vi "RT_Control_Adrian_Microphones+Angles+Force_NoPower.vi"(10 "rt fifo":refnum<k33>, 11 "Parameters":T1={"N_chan"=0, "Input Rate (Hz)"=0.0, "Acq Time (s)"=0.0, "NumOfWarmupIters"=0, "Size fifo"=0, "Period NCL (ms)"=0, "Timeout fifo Read"=0, "Size Sent Array"=0, "Output offsets"=[], "Input offsets"=[0.0, 0.0, 0.0, 0.0, 0.0, 0.0, 0.0, 0.0]}) -> (0 "error out":errorcluster, 1 "Total Iterations":i64, 2 "Delayed Cycles":dbl)   [LabVIEW 2021]
uses:
  parametersRT.ctl
  <vilib>/DAQmx/write.llb/DAQmx Write (Analog 1D DBL NChan 1Samp).vi
  <vilib>/DAQmx/read.llb/DAQmx Read (Analog 1D DBL NChan 1Samp).vi
  <vilib>/Analysis/baseanly.llb/A x Vector.vi
  <vilib>/DAQmx/read.llb/DAQmx Read (Digital 2D U32 NChan NSamp).vi
  <vilib>/Analysis/baseanly.llb/Mean (DBL).vi
  <vilib>/DAQmx/configure/timing.llb/DAQmx Timing (Sample Clock).vi
  <vilib>/DAQmx/miscellaneous.llb/DAQmx Fill In Error Info.vi
  <resource>/objmgr/daqmx.rc
  <vilib>/Analysis/NI_AALBase.lvlib
panel:
  out "output array":dbl[](array[numeric])
  out "data 2":u32[][](array[numeric])
  out "Encoder Raw Outputs":dbl[][](array[numeric])
  out "Encoder Mean Outputs":dbl[](array[numeric])
  in  "Zero Angle":dbl[](array[numeric])=[-16.79, 2.64, -15.0, 3.7]
  in  "source 2":tag
  in  "source":tag
  out "A x Vector":dbl[](array[numeric]) format="%.2f"
  in  "Unbias":bool
  out "Bias Voltages":dbl[][](array[numeric])=[[-0.0710179470114859, -0.17463349299050945, -0.11016159714741332, 0.026018829634351103, 0.12897648926553976, 0.08259620236774425]]
  out "Bias Vector":dbl[](array[numeric])=[-0.0710179470114859, -0.17463349299050945, -0.11016159714741332, 0.026018829634351103, 0.12897648926553976, 0.08259620236774425]
  in  "Bias":bool
  out "Voltages":dbl[][](array[numeric])=[[-0.07200476171213811, -0.17430455474177844, -0.11114841186574954, 0.027005644288728526, 0.12535816905124034, 0.08062257311350753], [-0.07233369994578917, -0.17397561649309423, -0.11147735010529275, 0.027334582506747616, 0.1263449836558195, 0.08160938774087402], [-0.0716758234785372, -0.17463349299050945, -0.11147735010529275, 0.026676706070656076, 0.1260160454543497, 0.08062257311350753], [-0.07200476171213811, -0.1749624312392873, -0.1118062883448848, 0.026676706070656076, 0.1256871072528233, 0.08029363490427514], [-0.07200476171213811, -0.17430455474177844, -0.11213522658452575, 0.026676706070656076, 0.12535816905124034, 0.08029363490427514], [-0.07233369994578917, -0.1749624312392873, -0.11147735010529275, 0.027334582506747616, 0.1260160454543497, 0.08062257311350753], [-0.07200476171213811, -0.17397561649309423, -0.11147735010529275, 0.027005644288728526, 0.1260160454543497, 0.08029363490427514], [-0.07200476171213811, -0.17463349299050945, -0.1118062883448848, 0.027005644288728526, 0.1260160454543497, 0.08062257311350753], [-0.07233369994578917, -0.17397561649309423, -0.11114841186574954, 0.027334582506747616, 0.1263449836558195, 0.08062257311350753], [-0.07233369994578917, -0.17463349299050945, -0.1118062883448848, 0.026676706070656076, 0.1256871072528233, 0.08029363490427514], [-0.07200476171213811, -0.17463349299050945, -0.11213522658452575, 0.027334582506747616, 0.1256871072528233, 0.08062257311350753], [-0.07233369994578917, -0.17463349299050945, -0.1118062883448848, 0.027005644288728526, 0.1256871072528233, 0.08029363490427514], [-0.07200476171213811, -0.17463349299050945, -0.1118062883448848, 0.027334582506747616, 0.1260160454543497, 0.08029363490427514], [-0.0716758234785372, -0.17430455474177844, -0.11147735010529275, 0.027334582506747616, 0.1263449836558195, 0.08128044953180698], [-0.07200476171213811, -0.17463349299050945, -0.11114841186574954, 0.027005644288728526, 0.1263449836558195, 0.08029363490427514], [-0.07266263817949037, -0.17430455474177844, -0.11213522658452575, 0.027005644288728526, 0.1256871072528233, 0.08029363490427514], [-0.07233369994578917, -0.17463349299050945, -0.1118062883448848, 0.027334582506747616, 0.1263449836558195, 0.08128044953180698], [-0.07200476171213811, -0.17397561649309423, -0.1118062883448848, 0.026676706070656076, 0.1260160454543497, 0.08029363490427514], [-0.07233369994578917, -0.17397561649309423, -0.11147735010529275, 0.027334582506747616, 0.1263449836558195, 0.08128044953180698], [-0.0716758234785372, -0.17397561649309423, -0.11147735010529275, 0.027334582506747616, 0.1256871072528233, 0.08029363490427514], [-0.07200476171213811, -0.17430455474177844, -0.1118062883448848, 0.027334582506747616, 0.1263449836558195, 0.08095151132268481], [-0.07266263817949037, -0.17463349299050945, -0.1118062883448848, 0.026676706070656076, 0.1260160454543497, 0.08029363490427514], [-0.07200476171213811, -0.1736466782444569, -0.1118062883448848, 0.027005644288728526, 0.12535816905124034, 0.08095151132268481], [-0.07233369994578917, -0.1749624312392873, -0.11147735010529275, 0.027005644288728526, 0.1263449836558195, 0.08062257311350753], [-0.07200476171213811, -0.1736466782444569, -0.11114841186574954, 0.02766352072471333, 0.1263449836558195, 0.08062257311350753], [-0.07200476171213811, -0.17463349299050945, -0.1118062883448848, 0.027005644288728526, 0.1256871072528233, 0.08029363490427514], [-0.07266263817949037, -0.17430455474177844, -0.11213522658452575, 0.027334582506747616, 0.1260160454543497, 0.08062257311350753], [-0.07200476171213811, -0.17430455474177844, -0.11147735010529275, 0.02766352072471333, 0.1263449836558195, 0.08062257311350753], [-0.07200476171213811, -0.1749624312392873, -0.11213522658452575, 0.027334582506747616, 0.1260160454543497, 0.08062257311350753], [-0.07233369994578917, -0.17430455474177844, -0.11147735010529275, 0.027334582506747616, 0.1260160454543497, 0.08029363490427514], [-0.07233369994578917, -0.17397561649309423, -0.1118062883448848, 0.027334582506747616, 0.1263449836558195, 0.08062257311350753], [-0.0716758234785372, -0.17397561649309423, -0.11213522658452575, 0.027334582506747616, 0.1260160454543497, 0.07996469669498764], [-0.07266263817949037, -0.17430455474177844, -0.1118062883448848, 0.02766352072471333, 0.1263449836558195, 0.08062257311350753], [-0.07266263817949037, -0.17430455474177844, -0.1118062883448848, 0.027334582506747616, 0.1256871072528233, 0.08029363490427514], [-0.07200476171213811, -0.17463349299050945, -0.1118062883448848, 0.026676706070656076, 0.12535816905124034, 0.07963575848564507], [-0.07233369994578917, -0.17397561649309423, -0.11114841186574954, 0.02766352072471333, 0.1263449836558195, 0.08062257311350753], [-0.07266263817949037, -0.1749624312392873, -0.11213522658452575, 0.026676706070656076, 0.12535816905124034, 0.07963575848564507], [-0.07233369994578917, -0.17463349299050945, -0.1118062883448848, 0.027005644288728526, 0.1256871072528233, 0.07996469669498764], [-0.07299157641324171, -0.17463349299050945, -0.11213522658452575, 0.026676706070656076, 0.1260160454543497, 0.08029363490427514], [-0.07233369994578917, -0.17430455474177844, -0.11147735010529275, 0.027334582506747616, 0.12667392185723272, 0.08095151132268481], [-0.07200476171213811, -0.1736466782444569, -0.11147735010529275, 0.02766352072471333, 0.1263449836558195, 0.08062257311350753], [-0.07233369994578917, -0.17397561649309423, -0.1118062883448848, 0.026676706070656076, 0.1260160454543497, 0.07996469669498764], [-0.07233369994578917, -0.17463349299050945, -0.11213522658452575, 0.027005644288728526, 0.1260160454543497, 0.08029363490427514], [-0.07200476171213811, -0.17331773999586642, -0.11081947362625524, 0.02766352072471333, 0.12667392185723272, 0.08095151132268481], [-0.07233369994578917, -0.17397561649309423, -0.1118062883448848, 0.02766352072471333, 0.1260160454543497, 0.08029363490427514], [-0.07266263817949037, -0.17463349299050945, -0.11213522658452575, 0.02766352072471333, 0.1260160454543497, 0.08128044953180698], [-0.07200476171213811, -0.17397561649309423, -0.11147735010529275, 0.02766352072471333, 0.1263449836558195, 0.08095151132268481], [-0.07200476171213811, -0.17430455474177844, -0.1118062883448848, 0.027334582506747616, 0.1263449836558195, 0.08095151132268481], [-0.0716758234785372, -0.17463349299050945, -0.1118062883448848, 0.027005644288728526, 0.1263449836558195, 0.08095151132268481], [-0.07200476171213811, -0.17397561649309423, -0.1118062883448848, 0.027005644288728526, 0.1256871072528233, 0.08029363490427514], [-0.07233369994578917, -0.17430455474177844, -0.11147735010529275, 0.027334582506747616, 0.1263449836558195, 0.08095151132268481], [-0.0716758234785372, -0.1736466782444569, -0.11114841186574954, 0.027992458942625646, 0.12667392185723272, 0.08095151132268481], [-0.07200476171213811, -0.17397561649309423, -0.1118062883448848, 0.027334582506747616, 0.1263449836558195, 0.08029363490427514], [-0.07200476171213811, -0.17397561649309423, -0.11114841186574954, 0.027334582506747616, 0.1263449836558195, 0.08029363490427514], [-0.07233369994578917, -0.17397561649309423, -0.1118062883448848, 0.027334582506747616, 0.1260160454543497, 0.08029363490427514], [-0.07266263817949037, -0.17430455474177844, -0.11213522658452575, 0.026676706070656076, 0.1260160454543497, 0.08029363490427514], [-0.07233369994578917, -0.17397561649309423, -0.11213522658452575, 0.027334582506747616, 0.1263449836558195, 0.08062257311350753], [-0.07233369994578917, -0.17463349299050945, -0.11213522658452575, 0.027334582506747616, 0.1260160454543497, 0.08029363490427514], [-0.07200476171213811, -0.17331773999586642, -0.11147735010529275, 0.027334582506747616, 0.1263449836558195, 0.08029363490427514], [-0.07233369994578917, -0.1749624312392873, -0.11213522658452575, 0.026676706070656076, 0.1260160454543497, 0.08029363490427514], [-0.07233369994578917, -0.17463349299050945, -0.1118062883448848, 0.027005644288728526, 0.1260160454543497, 0.08029363490427514], [-0.07233369994578917, -0.17397561649309423, -0.1118062883448848, 0.027334582506747616, 0.12667392185723272, 0.08062257311350753], [-0.07200476171213811, -0.17430455474177844, -0.11147735010529275, 0.027334582506747616, 0.1260160454543497, 0.07996469669498764], [-0.07233369994578917, -0.17430455474177844, -0.1118062883448848, 0.027334582506747616, 0.12667392185723272, 0.08095151132268481], [-0.0716758234785372, -0.17430455474177844, -0.11147735010529275, 0.026676706070656076, 0.1263449836558195, 0.08029363490427514], [-0.07266263817949037, -0.17430455474177844, -0.11147735010529275, 0.027005644288728526, 0.1263449836558195, 0.07996469669498764], [-0.07266263817949037, -0.1749624312392873, -0.11246416482421552, 0.026676706070656076, 0.1263449836558195, 0.08029363490427514], [-0.07266263817949037, -0.17397561649309423, -0.1118062883448848, 0.027334582506747616, 0.1263449836558195, 0.08029363490427514], [-0.0716758234785372, -0.1736466782444569, -0.11147735010529275, 0.02766352072471333, 0.1263449836558195, 0.08062257311350753], [-0.07233369994578917, -0.17397561649309423, -0.1118062883448848, 0.027334582506747616, 0.1263449836558195, 0.08095151132268481], [-0.07233369994578917, -0.17430455474177844, -0.1118062883448848, 0.027334582506747616, 0.1260160454543497, 0.08062257311350753], [-0.0716758234785372, -0.17331773999586642, -0.11081947362625524, 0.027992458942625646, 0.12700286005858935, 0.08062257311350753], [-0.07233369994578917, -0.17397561649309423, -0.11213522658452575, 0.027005644288728526, 0.1263449836558195, 0.08029363490427514], [-0.07233369994578917, -0.17463349299050945, -0.11147735010529275, 0.027005644288728526, 0.1260160454543497, 0.08029363490427514], [-0.07266263817949037, -0.1736466782444569, -0.11147735010529275, 0.02766352072471333, 0.12667392185723272, 0.08029363490427514], [-0.07200476171213811, -0.17463349299050945, -0.11213522658452575, 0.026676706070656076, 0.1260160454543497, 0.07996469669498764], [-0.07266263817949037, -0.17430455474177844, -0.11213522658452575, 0.027005644288728526, 0.1263449836558195, 0.08062257311350753], [-0.07200476171213811, -0.17397561649309423, -0.11147735010529275, 0.02766352072471333, 0.1263449836558195, 0.08062257311350753], [-0.07200476171213811, -0.17397561649309423, -0.1118062883448848, 0.027005644288728526, 0.1263449836558195, 0.08029363490427514], [-0.07233369994578917, -0.17430455474177844, -0.11213522658452575, 0.027005644288728526, 0.1263449836558195, 0.08062257311350753], [-0.07233369994578917, -0.1736466782444569, -0.11114841186574954, 0.027334582506747616, 0.12667392185723272, 0.08062257311350753], [-0.07233369994578917, -0.17430455474177844, -0.1118062883448848, 0.027334582506747616, 0.1260160454543497, 0.08029363490427514], [-0.07266263817949037, -0.17529136948811197, -0.11279310306395414, 0.026676706070656076, 0.1263449836558195, 0.08029363490427514], [-0.07233369994578917, -0.17397561649309423, -0.11147735010529275, 0.027005644288728526, 0.12667392185723272, 0.08062257311350753], [-0.07200476171213811, -0.17430455474177844, -0.1118062883448848, 0.027334582506747616, 0.1263449836558195, 0.07996469669498764], [-0.07233369994578917, -0.17463349299050945, -0.11246416482421552, 0.027005644288728526, 0.1256871072528233, 0.07996469669498764], [-0.07266263817949037, -0.17430455474177844, -0.1118062883448848, 0.026676706070656076, 0.1260160454543497, 0.07996469669498764], [-0.07266263817949037, -0.17463349299050945, -0.1118062883448848, 0.027005644288728526, 0.1260160454543497, 0.08062257311350753], [-0.07266263817949037, -0.17397561649309423, -0.1118062883448848, 0.02766352072471333, 0.1263449836558195, 0.07996469669498764], [-0.07233369994578917, -0.17463349299050945, -0.1118062883448848, 0.027005644288728526, 0.1260160454543497, 0.08062257311350753], [-0.0716758234785372, -0.17397561649309423, -0.11114841186574954, 0.02766352072471333, 0.12667392185723272, 0.08095151132268481], [-0.07200476171213811, -0.17430455474177844, -0.11147735010529275, 0.027005644288728526, 0.1260160454543497, 0.08029363490427514], [-0.07200476171213811, -0.17397561649309423, -0.11114841186574954, 0.027992458942625646, 0.12700286005858935, 0.08128044953180698], [-0.07134688524498646, -0.17397561649309423, -0.1118062883448848, 0.027005644288728526, 0.1263449836558195, 0.07996469669498764], [-0.07266263817949037, -0.17463349299050945, -0.11213522658452575, 0.026676706070656076, 0.1256871072528233, 0.07996469669498764], [-0.07266263817949037, -0.17430455474177844, -0.11147735010529275, 0.027334582506747616, 0.12667392185723272, 0.08062257311350753], [-0.0716758234785372, -0.17463349299050945, -0.1118062883448848, 0.026676706070656076, 0.12667392185723272, 0.08029363490427514], [-0.07233369994578917, -0.17397561649309423, -0.1118062883448848, 0.027334582506747616, 0.1263449836558195, 0.08062257311350753], [-0.07233369994578917, -0.17463349299050945, -0.1118062883448848, 0.027005644288728526, 0.1260160454543497, 0.08029363490427514], [-0.07233369994578917, -0.17397561649309423, -0.11213522658452575, 0.027334582506747616, 0.1263449836558195, 0.08062257311350753]]
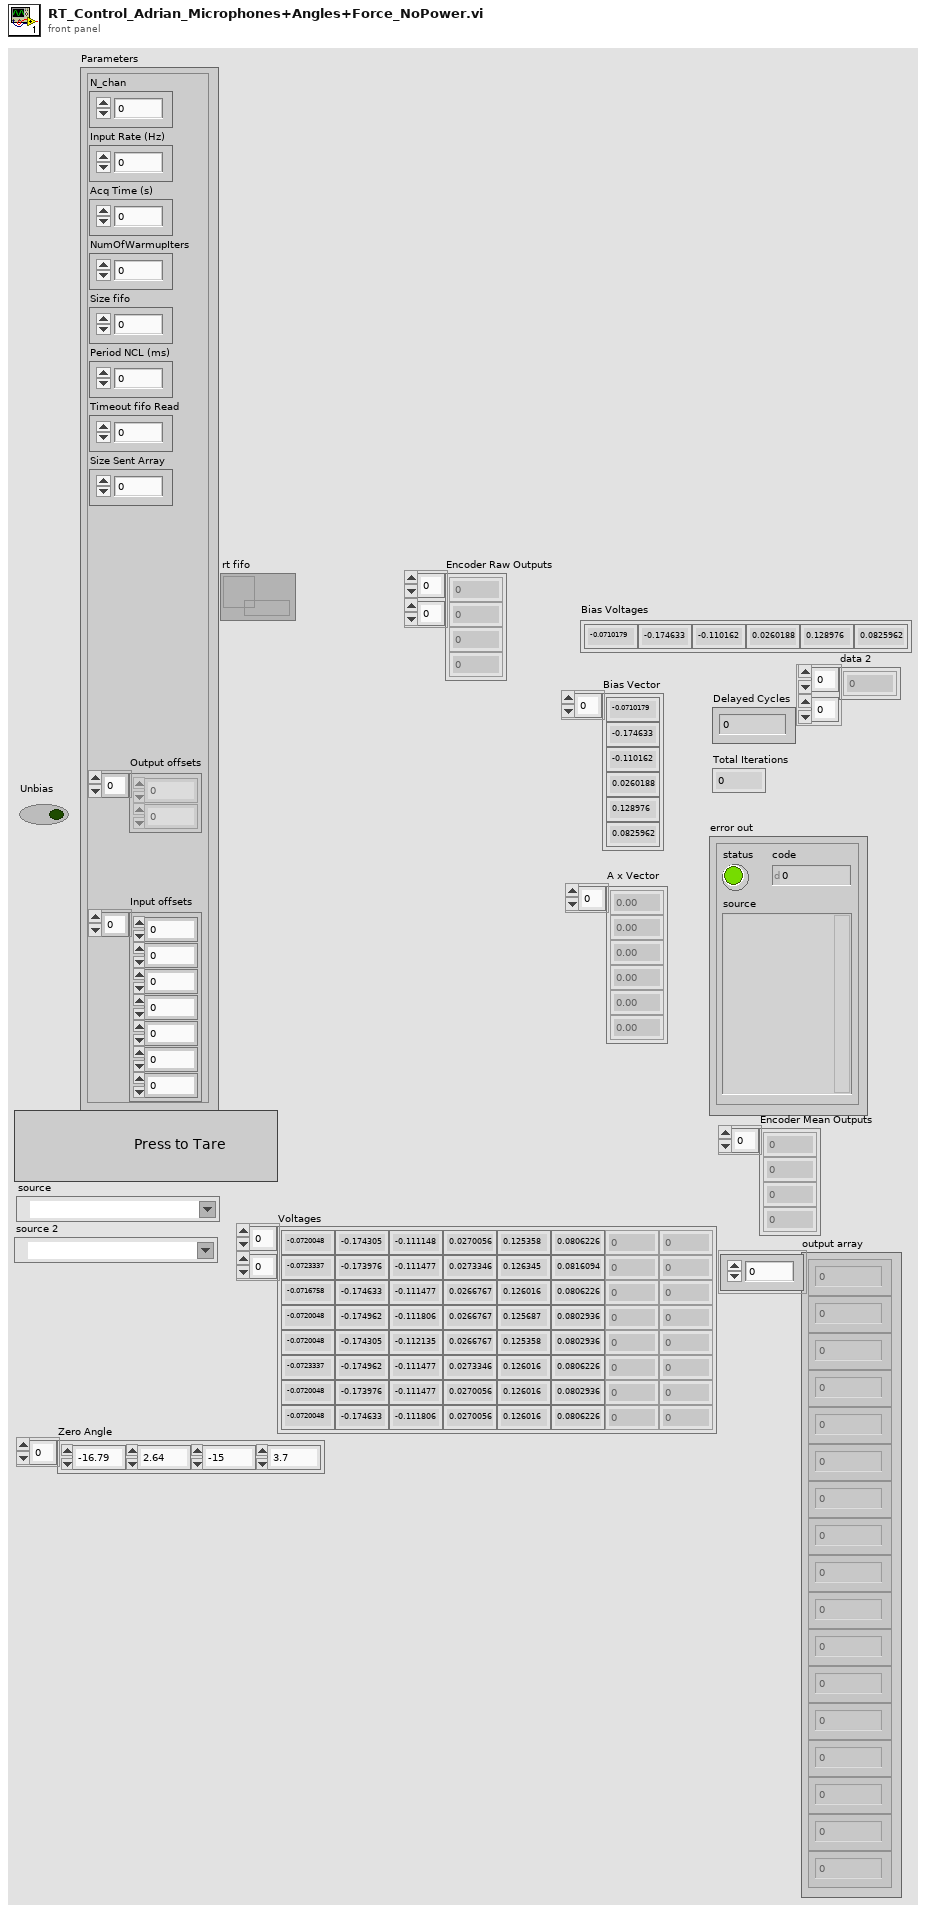
[diagram p1: front panel]
types:
  T1 = typedef "parametersRT.ctl" = cluster{"N_chan":u32, "Input Rate (Hz)":dbl, "Acq Time (s)":dbl, "NumOfWarmupIters":u32, "Size fifo":u32, "Period NCL (ms)":i64, "Timeout fifo Read":i32, "Size Sent Array":i32, "Output offsets":dbl[], "Input offsets":dbl[]}
  T2 = cluster{"Csn task out":refnum<k21>, "CLK task out":refnum<k21>, "D0 task out":refnum<k21>}
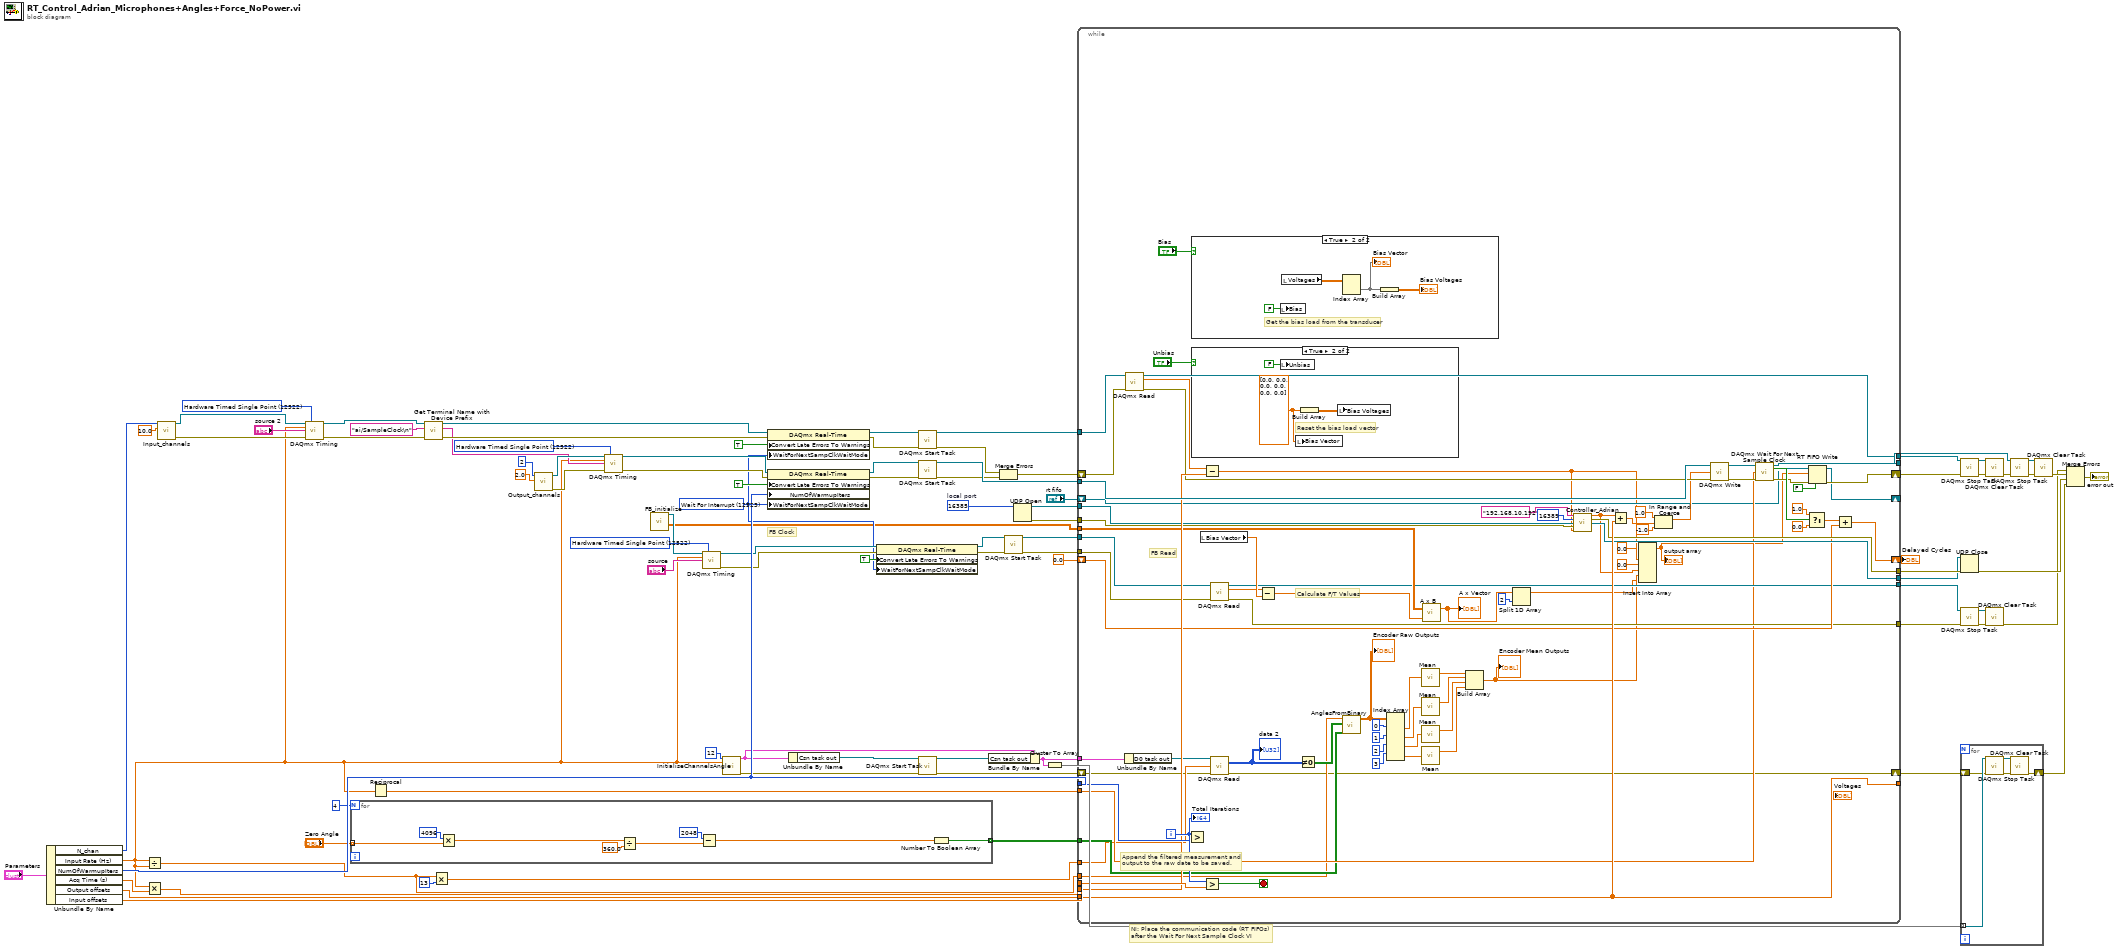
[diagram p0: block diagram]
diagram:
  w48 = 12522 items=["Finite Samples"=10178, "Continuous Samples"=10123, "Hardware Timed Single Point"=12522] ("sample mode")
  w59 = u16 16385  # local port
  w66 = 12522 items=["Finite Samples"=10178, "Continuous Samples"=10123, "Hardware Timed Single Point"=12522] ("sample mode")
  w43 = 12523 items=["Wait For Interrupt"=12523, "Poll"=12524, "Yield"=12525] ("WaitForNextSampClkWaitMode")
  w89 = 12522 items=["Finite Samples"=10178, "Continuous Samples"=10123, "Hardware Timed Single Point"=12522] ("sample mode")
  # "FB Clock"
  # "NI: Place the communication code (RT FIFOs) \nafter the Wait For Next Sample Clock VI"
  n1 = Unbundle By Name("Parameters") -> ("N_chan"=w75:u32, "Input Rate (Hz)"=w10:dbl, "NumOfWarmupIters"=w76:u32, "Acq Time (s)"=w83:dbl, "Output offsets"=w74:dbl[], "Input offsets"=w73:dbl[])
  n2 = Divide(x=w10, y=w10) -> (x/y=w8:dbl)
  n3 = Multiply(x=w10, y=w83) -> (x*y=w53:dbl)
  n4 = call "Input_channels.vi"("Range"=10.0, "nchan"=w75) -> ("error out"=w68:errorcluster, "Refnum out"=w67:refnum<k21>)  [unwired: 8 in]
  n5 = call-poly <vilib>:"DAQmx Timing.vi"("task/channels in"=w67, "sample mode"=w66, "rate"=w10, "source"="source 2", "error in"=w68) -> ("task out"=w36:refnum<k21>, "error out"=w34:errorcluster)  [unwired: 9 in]
  n6 = for {
    N: 4 -> [_]
    tunnel: [w94] -> w9 mode=indexing
    tunnel: "Zero Angle" -> [w97] mode=indexing
    n7 = Multiply(x=4096, y=w97) -> (x*y=w98:dbl)
    n8 = Divide(x=w98, y=360.0) -> (x/y=w92:dbl)
    n9 = Subtract(x=2048, y=w92) -> (x-y=w91:dbl)
    n10 = Number To Boolean Array(number=w91) -> (Boolean array=w94:bool[])
  }
  n11 = Reciprocal(x=w10) -> (1/x=w88:dbl)
  n12 = call "Get Terminal Name with Device Prefix.vi"("error in (no error)"=w34, "Local Terminal Name"="ai/SampleClock\n", "task/channels in"=w36) -> ("error out"=w33:errorcluster, "Terminal Name with Device Prefix"=w32:tag, "task out"=w35:refnum<k21>)  [unwired: 6 in]
  n13 = Multiply(x=w8, y=13) -> (x*y=w6:dbl)
  n14 = call "Output_channels.vi"("Range"=2.0 ("Maximum Value"), "nchan"=2) -> ("error out"=w80:errorcluster, "Refnum out"=w79:refnum<k21>)  [unwired: 8 in]
  n15 = call-poly <vilib>:"DAQmx Timing.vi"("task/channels in"=w79, "sample mode"=w89, "rate"=w10, "source"=w32, "error in"=w80) -> ("task out"=w87:refnum<k21>, "error out"=w86:errorcluster)  [unwired: 9 in]
  n16 = call "FB_initialize.vi"() -> ("Transformed Calibration Matrix"=w40:dbl[][], "FB out"=w44:refnum<k21>)  [unwired: 9 in, 1 out]
  n17 = call-poly <vilib>:"DAQmx Timing.vi"("task/channels in"=w44, "sample mode"=w48, "rate"=w10, "source"="source") -> ("task out"=w50:refnum<k21>, "error out"=w49:errorcluster)  [unwired: 10 in]
  n18 = call "InitialiseChannelsAngle.vi"("Number of data bits"=12, "Fs"=w10) -> ("output cluster"=w11:T2, "error out"=w12:errorcluster)  [unwired: 12 in]
  n19 = property class="DAQmx Real-Time"(reference=w35, error in=w33, "Convert Late Errors To Warnings"=TRUE, "WaitForNextSampClkWaitMode"=w43) -> (reference out=w63:refnum<k21>, error out=w62:errorcluster)
  n20 = property class="DAQmx Real-Time"(reference=w87, error in=w86, "Convert Late Errors To Warnings"=TRUE, "NumOfWarmupIters"=w76, "WaitForNextSampClkWaitMode"=w43) -> (reference out=w84:refnum<k21>, error out=w70:errorcluster)
  n21 = Unbundle By Name(w11) -> ("Csn task out"=w16:refnum<k21>)
  n22 = property class="DAQmx Real-Time"(reference=w50, error in=w49, "Convert Late Errors To Warnings"=TRUE ("ConvLateErrorsToWarnings"), "WaitForNextSampClkWaitMode"=w43) -> (reference out=w45:refnum<k21>, error out=w46:errorcluster)
  n23 = call <vilib>:"DAQmx Start Task.vi"("task/channels in"=w63, "error in"=w62) -> ("task out"=w82:refnum<k21>, "error out"=w61:errorcluster)  [unwired: 12 in]
  n24 = call <vilib>:"DAQmx Start Task.vi"("task/channels in"=w84, "error in"=w70) -> ("task out"=w81:refnum<k21>, "error out"=w69:errorcluster)  [unwired: 12 in]
  n25 = call <vilib>:"DAQmx Start Task.vi"("task/channels in"=w16, "error in"=w12) -> ("task out"=w15:refnum<k21>, "error out"=w3:errorcluster)  [unwired: 12 in]
  n26 = Bundle By Name(cluster=w11, "Csn task out"=w15) -> (w7:T2)
  n27 = Merge Errors(w61, w69) -> (w60:errorcluster)
  n28 = call <vilib>:"DAQmx Start Task.vi"("task/channels in"=w45, "error in"=w46) -> ("task out"=w42:refnum<k21>, "error out"=w41:errorcluster)  [unwired: 12 in]
  n29 = UDP Open(11:w59) -> (port=w57:refnum<k16>, 0:w58:errorcluster)  [unwired: 4 in, 1 out]
  n30 = Cluster To Array(cluster=w7) -> (array=w5:refnum<k21>[])
  n31 = while {
    shift-right: [w111] -> w25
    shift-left: w60 -> [w164]
    shift-right: [w173] -> w90
    shift-left: 0.0 ("f") -> [w152]
    tunnel: w88 -> [w135]
    tunnel: w53 -> [w171]
    tunnel: w81 -> [w170]
    tunnel: [w165] -> w24
    tunnel: w82 -> [w166]
    tunnel: [w137] -> w20
    tunnel: w76 -> [w168]
    tunnel: w74 -> [w160]
    tunnel: [w160] -> _
    tunnel: w73 -> [w167]
    tunnel: w58 -> [w158]
    tunnel: w57 -> [w157]
    tunnel: [w156] -> w56
    tunnel: [w155] -> w55
    tunnel: w42 -> [w151]
    tunnel: w41 -> [w150]
    tunnel: w40 -> [w145]
    tunnel: [w144] -> w30
    tunnel: [w143] -> w28
    tunnel: w9 -> [w118]
    tunnel: w8 -> [w117]
    tunnel: w7 -> [w116]
    tunnel: w6 -> [w115]
    shift-right: [w114] -> w4
    shift-left: w3 -> [w113]
    shift-right: [w103] -> _
    shift-left: "rt fifo" -> [w102]
    i -> [w169]
    stop <- w172 stop-if-true
    # "Calculate F/T Values"
    # "FB Read"
    # "Append the filtered measurement and \noutput to the raw date to be saved."
    n32 = Unbundle By Name(w116) -> ("D0 task out"=w134:refnum<k21>)
    n33 = call-poly <vilib>:"DAQmx Read.vi"("task/channels in"=w166, "error in"=w164) -> ("task out"=w165:refnum<k21>, "data"=w99:dbl[], "error out"=w163:errorcluster)  [unwired: 11 in]
    n34 = Greater?(x=w169, y=w168) -> ()  [unwired: 1 out]
    n35 = case shown="True" "Bias" {
      frame False {
      }
      frame True {
        # "Get the bias load from the transducer"
        n36 = local write "Bias"(FALSE) -> ()
        n37 = local read "Voltages"() -> (w183:dbl[][])
        n38 = Index Array(array=w183) -> (element=w180:dbl[])  [unwired: 2 in]
        "Bias Vector" <- w180
        n39 = Build Array(w180) -> (→"Bias Voltages":dbl[][])
      }
    }
    n40 = case shown="True" "Unbias" {
      frame False {
      }
      frame True {
        w178 = dbl[] [0.0, 0.0, 0.0, 0.0, 0.0, 0.0]
        # "Reset the bias load vector"
        n41 = local write "Unbias"(FALSE) -> ()
        n42 = local write "Bias Vector"(w178) -> ()
        n43 = Build Array(w178) -> (w177:dbl[][])
        n44 = local write "Bias Voltages"(w177) -> ()
      }
    }
    n45 = local read "Bias Vector"() -> (w147:dbl[])
    n46 = Subtract(x=w99, y=w167) -> (x-y=w100:dbl[])
    n47 = Greater?(x=w169, y=w171) -> (0:w172:bool)
    n48 = call-poly <vilib>:"DAQmx Read.vi"("task/channels in"=w151, "error in"=w150) -> ("task out"=w144:refnum<k21>, "data"=w101:dbl[], "error out"=w143:errorcluster)  [unwired: 11 in]
    n49 = call-poly <vilib>:"DAQmx Read.vi"("task/channels in"=w134, "number of samples per channel"=w115, "error in"=w113) -> ("data"=w133:u32[][], "error out"=w114:errorcluster)  [unwired: 10 in, 1 out]
    "data 2" <- w133
    n50 = Subtract(x=w101, y=w147) -> (x-y=w146:dbl[])
    n51 = Not Equal To 0?(x=w133) -> (x != 0?=w119:bool[][])
    n52 = call "AnglesFromBinary.vi"("Binary Offset"=w118, "Array"=w119, "Buffer Length"=w117) -> ("Unwrapped Phase"=w132:dbl[][])  [unwired: 8 in]
    "Encoder Raw Outputs" <- w132
    n53 = Index Array(array=w132, index (row) #1=0 ("index (row)"), index (row) #2=1 ("index (row)"), index (row) #3=2 ("index (row)"), index (row) #4=3 ("index (row)")) -> (element #1=w127:dbl[], element #2=w126:dbl[], element #3=w125:dbl[], element #4=w124:dbl[])  [unwired: 4 in]
    n54 = call-poly <vilib>:"Mean.vi"("X"=w127) -> ("mean"=w120:dbl)  [unwired: 1 out]
    n55 = call-poly <vilib>:"Mean.vi"("X"=w126) -> ("mean"=w121:dbl)  [unwired: 1 out]
    n56 = call-poly <vilib>:"Mean.vi"("X"=w125) -> ("mean"=w122:dbl)  [unwired: 1 out]
    n57 = call-poly <vilib>:"Mean.vi"("X"=w124) -> ("mean"=w123:dbl)  [unwired: 1 out]
    n58 = call-poly <vilib>:"A x B.vi"("Vector"=w146, "A"=w145) -> ("A x Vector"=w141:dbl[])  [unwired: 1 out]
    "A x Vector" <- w141
    n59 = Build Array(w120, w121, w122, w123) -> (w106:dbl[])
    "Encoder Mean Outputs" <- w106
    n60 = Split 1D Array(array=w141, index=2) -> (first subarray=w105:dbl[])  [unwired: 1 out]
    n61 = call "Controller_Adrian.vi"("name 2"="192.168.10.192", "port or service name"=u16 16389, "connection ID"=w157, "error in (no error)"=w158, "x"=w100) -> ("*(type *) &x"=w107:dbl[], "error out"=w156:errorcluster, "connection ID out"=w155:refnum<k16>)  [unwired: 8 in]
    n62 = Add(x=w107, y=w160) -> (x+y=w140:dbl[])
    n63 = Insert Into Array(array=w100, new element #1=0.0 ("new element/subarray"), new element #2=0.0 ("new element/subarray"), new element #3=w107, new element #4=w106, new element #5=w105) -> (w104:dbl[])  [unwired: 1 in]
    "output array" <- w104
    n64 = In Range and Coerce(upper limit=1.0, x=w140, lower limit=-1.0) -> (coerced(x)=w159:dbl[])  [unwired: 1 out]
    n65 = call-poly <vilib>:"DAQmx Write.vi"("task/channels in"=w170, "data"=w159, "error in"=w163) -> ("task out"=w138:refnum<k21>, "error out"=w139:errorcluster)  [unwired: 10 in, 1 out]
    n66 = call <vilib>:"DAQmx Wait For Next Sample Clock.vi"("task/channels in"=w138, "timeout (sec)"=w135, "error in"=w139) -> ("task out"=w137:refnum<k21>, "is late?"=w136:bool, "error out"=w110:errorcluster)  [unwired: 10 in]
    n67 = Select(t=1.0, s=w136, f=0.0) -> (s? t:f=w174:dbl)
    n68 = RT FIFO Write(0:w102, 1:w104, 3:w110, 5:FALSE ("overwrite on timeout (T)")) -> (8:w103:refnum<k33>, 11:w111:errorcluster)  [unwired: 1 in, 2 out]
    n69 = Add(x=w174, y=w152) -> (x+y=w173:dbl)
    "Total Iterations" <- w169
  }
  "Delayed Cycles" <- w90
  n70 = call <vilib>:"DAQmx Stop Task.vi"("task/channels in"=w24, "error in"=w25) -> ("task out"=w23:refnum<k21>, "error out"=w26:errorcluster)  [unwired: 12 in]
  n71 = UDP Close(connection ID=w55, 8:w56) -> (error out=w54:errorcluster)  [unwired: 1 out]
  n72 = call <vilib>:"DAQmx Stop Task.vi"("task/channels in"=w30, "error in"=w28) -> ("task out"=w29:refnum<k21>, "error out"=w27:errorcluster)  [unwired: 12 in]
  n73 = for {
    tunnel: w5 -> [w188] mode=indexing
    shift-right: [w184] -> w2
    shift-left: w4 -> [w186]
    n74 = call <vilib>:"DAQmx Stop Task.vi"("task/channels in"=w188, "error in"=w186) -> ("task out"=w187:refnum<k21>, "error out"=w185:errorcluster)  [unwired: 12 in]
    n75 = call <vilib>:"DAQmx Clear Task.vi"("task in"=w187, "error in"=w185) -> ("error out"=w184:errorcluster)  [unwired: 13 in]
  }
  n76 = call <vilib>:"DAQmx Clear Task.vi"("task in"=w23, "error in"=w26) -> ("error out"=w22:errorcluster)  [unwired: 13 in]
  n77 = call <vilib>:"DAQmx Clear Task.vi"("task in"=w29, "error in"=w27) -> ("error out"=w39:errorcluster)  [unwired: 13 in]
  n78 = call <vilib>:"DAQmx Stop Task.vi"("task/channels in"=w20, "error in"=w22) -> ("task out"=w19:refnum<k21>, "error out"=w21:errorcluster)  [unwired: 12 in]
  n79 = call <vilib>:"DAQmx Clear Task.vi"("task in"=w19, "error in"=w21) -> ("error out"=w72:errorcluster)  [unwired: 13 in]
  n80 = Merge Errors(w39, w72, w54, w2) -> (→"error out":errorcluster)
